vi "Copy Raw Data.vi"(8 "error in (no error)":errorcluster, 10 "new tdms file":refnum<k34>, 11 "original tdms file":refnum<k34>) -> (0 "error out":errorcluster, 3 "dup original tdms file":refnum<k34>)   [LabVIEW 2023]
doc: "Read raw data out from original file using standard read and write it to the new file with advanced synchronous write"
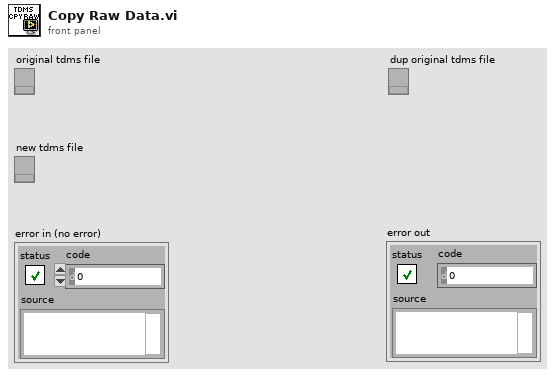
[diagram p1: front panel]
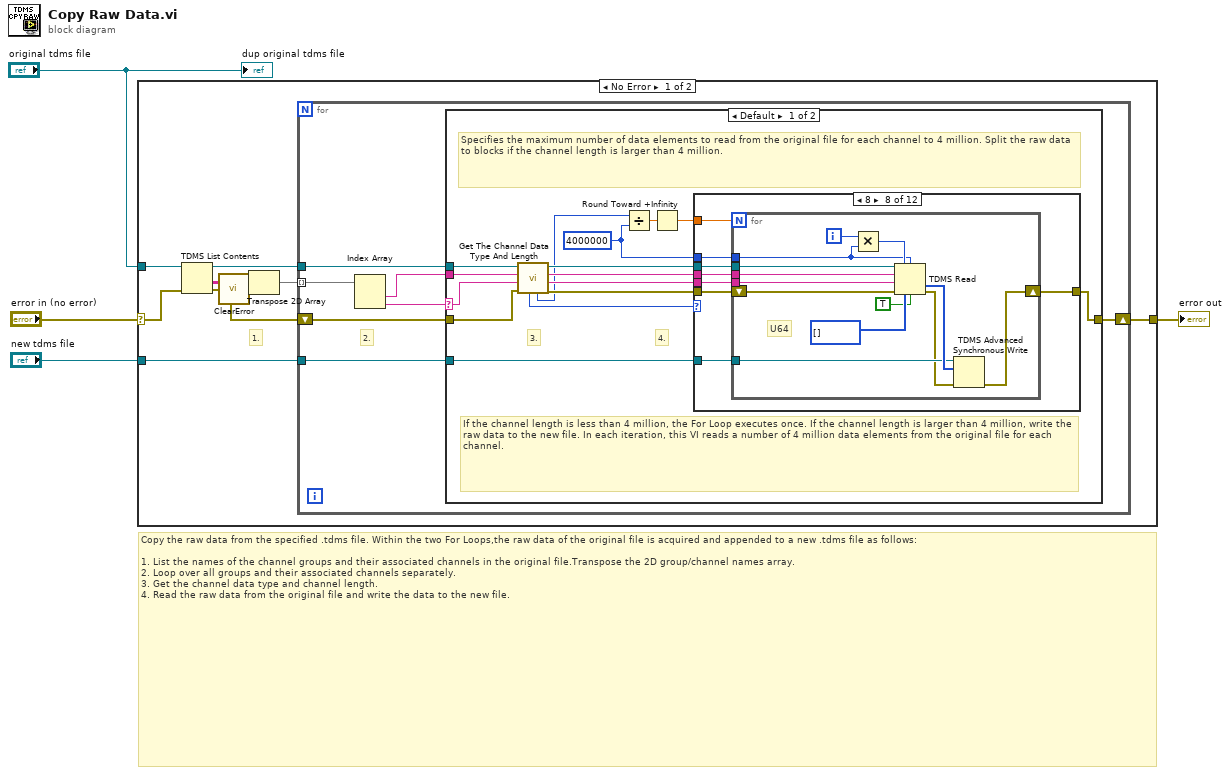
[diagram p0: block diagram]
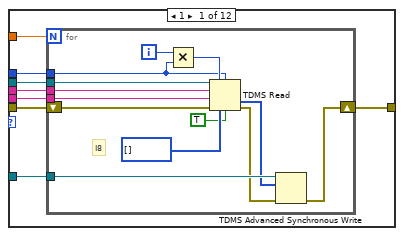
[diagram p2: hidden frame]
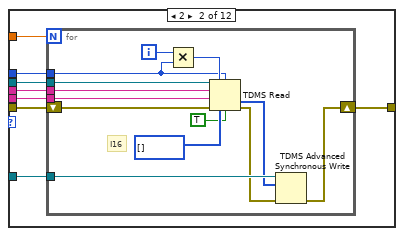
[diagram p3: hidden frame]
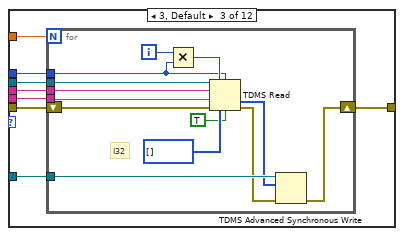
[diagram p4: hidden frame]
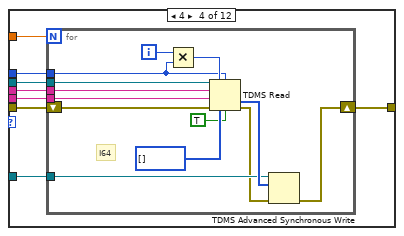
[diagram p5: hidden frame]
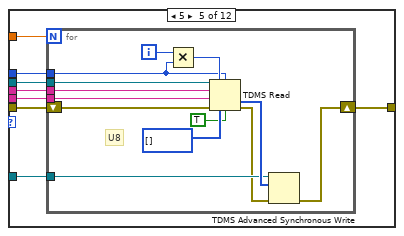
[diagram p6: hidden frame]
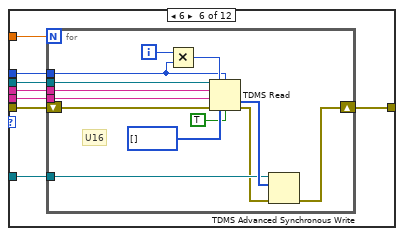
[diagram p7: hidden frame]
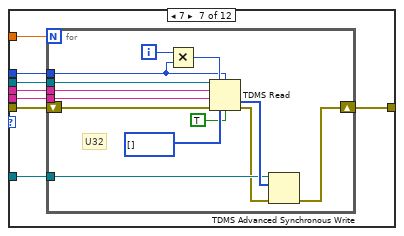
[diagram p8: hidden frame]
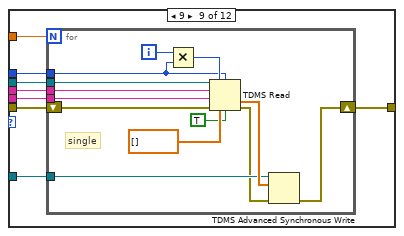
[diagram p9: hidden frame]
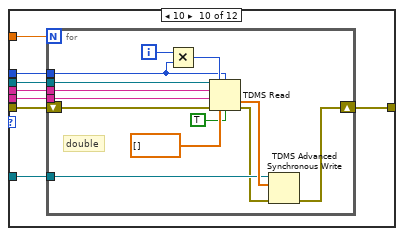
[diagram p10: hidden frame]
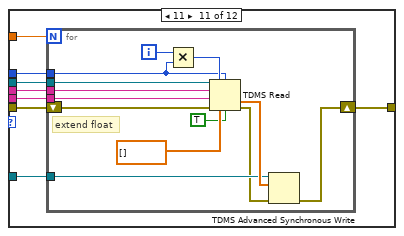
[diagram p11: hidden frame]
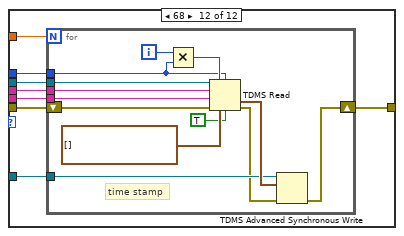
[diagram p12: hidden frame]
diagram:
  # "Copy the raw data from the specified .tdms file. Within the two For Loops,the raw data of the original file is acquired and appended to a new .tdms file as follows:\n\n1. List the names of the channel groups and their associated channels in the original file.Transpose the 2D group/channel names array.\n2. Loop over all groups and their associated channels separately.\n3. Get the channel data type and channel length.\n4. Read the raw data from the original file and write the data to the new file."
  n1 = case shown="No Error" "error in (no error)" {
    selector: "error in (no error)" -> [w7 w289]
    tunnel: "new tdms file" -> [w13 _]
    tunnel: [w12 w289] -> w2
    tunnel: "original tdms file" -> [w9 _]
    frame No Error {
      # "1."
      n2 = TDMS List Contents(4:w7, 7:w9) -> (0:w5:errorcluster, 1:w10:string[][], 3:w8:refnum<k34>)  [unwired: 1 in, 1 out]
      n3 = call <vilib>:"ClearError.vi"("error in (no error)"=w5) -> ("error out"=w6:errorcluster)
      n4 = Transpose 2D Array(2D array=w10) -> (transposed array=w11:string[][])
      n5 = for {
        shift-right: [w17] -> w12
        shift-left: w6 -> [w18]
        tunnel: w11 -> [w15] mode=indexing
        tunnel: w8 -> [w20]
        tunnel: w13 -> [w19]
        # "2."
        n6 = Index Array(array=w15) -> (element #1=w16:string, element #2=w14:string)  [unwired: 2 in]
        n7 = case shown="Default" w14 {
          selector: w14 -> [w21 _]
          tunnel: w20 -> [w35 _]
          tunnel: w19 -> [w34 _]
          tunnel: w18 -> [w33 w288]
          tunnel: [w31 w288] -> w17
          tunnel: w16 -> [w26 _]
          frame Default {
            w24 = 4000000 ("y")
            # "If the channel length is less than 4 million, the For Loop executes once. If the channel length is larger than 4 million, write the raw data to the new file. In each iteration, this VI reads a number of 4 million data elements from the original file for each channel."
            # "Specifies the maximum number of data elements to read from the original file for each channel to 4 million. Split the raw data to blocks if the channel length is larger than 4 million."
            # "4."
            # "3."
            n8 = call "Get The Channel Data Type And Length.vi"("error in (no error)"=w33, "channel name"=w21, "group name"=w26, "tdms file"=w35) -> ("error out"=w32:errorcluster, "dup channel name"=w27:string, "dup group name"=w28:string, "dup tdms file"=w30:refnum<k34>, "channel length"=w25:i32, "data type"=w29:i32)  [unwired: 2 in]
            n9 = Divide(x=w25, y=w24) -> (x/y=w23:dbl)
            n10 = Round Toward +Infinity(x=w23) -> (ceil(x): smallest int >= x=w22:dbl)
            n11 = case shown="8" w29 {
              tunnel: w30 -> [w41 w62 w83 w104 w125 w146 w167 w188 w209 w230 w251 w272]
              tunnel: w34 -> [w40 w61 w82 w103 w124 w145 w166 w187 w208 w229 w250 w271]
              tunnel: w28 -> [w39 w60 w81 w102 w123 w144 w165 w186 w207 w228 w249 w270]
              tunnel: w27 -> [w38 w59 w80 w101 w122 w143 w164 w185 w206 w227 w248 w269]
              tunnel: w22 -> [w43 w64 w85 w106 w127 w148 w169 w190 w211 w232 w253 w274]
              tunnel: w24 -> [w42 w63 w84 w105 w126 w147 w168 w189 w210 w231 w252 w273]
              tunnel: w32 -> [w37 w58 w79 w100 w121 w142 w163 w184 w205 w226 w247 w268]
              tunnel: [w36 w57 w78 w99 w120 w141 w162 w183 w204 w225 w246 w267] -> w31
              frame 1 {
                n12 = for {
                  N: w43 -> [_]
                  tunnel: w42 -> [w47]
                  tunnel: w39 -> [w53]
                  tunnel: w38 -> [w52]
                  shift-right: [w48] -> w36
                  shift-left: w37 -> [w50]
                  tunnel: w41 -> [w55]
                  tunnel: w40 -> [w54]
                  i -> [w51]
                  # "I8"
                  n13 = Multiply(x=w51, y=w47) -> (x*y=w56:i32)
                  n14 = TDMS Read(0:w55, 1:w56, 2:w47, 5:w53, 7:w52, 11:w50, 12:i8[] [], 13:TRUE ("return channels in file order? (F)")) -> (10:w46:i8[], 15:w49:errorcluster)  [unwired: 4 out]
                  n15 = TDMS Advanced Synchronous Write(8:w49, 10:w46, 11:w54) -> (0:w48:errorcluster)  [unwired: 1 out]
                }
              }
              frame 2 {
                n16 = for {
                  N: w64 -> [_]
                  tunnel: w63 -> [w68]
                  tunnel: w60 -> [w74]
                  tunnel: w59 -> [w73]
                  shift-right: [w69] -> w57
                  shift-left: w58 -> [w71]
                  tunnel: w62 -> [w76]
                  tunnel: w61 -> [w75]
                  i -> [w72]
                  # "I16"
                  n17 = Multiply(x=w72, y=w68) -> (x*y=w77:i32)
                  n18 = TDMS Read(0:w76, 1:w77, 2:w68, 5:w74, 7:w73, 11:w71, 12:i16[] [], 13:TRUE ("return channels in file order? (F)")) -> (10:w67:i16[], 15:w70:errorcluster)  [unwired: 4 out]
                  n19 = TDMS Advanced Synchronous Write(8:w70, 10:w67, 11:w75) -> (0:w69:errorcluster)  [unwired: 1 out]
                }
              }
              frame 3, Default {
                n20 = for {
                  N: w85 -> [_]
                  tunnel: w84 -> [w89]
                  tunnel: w81 -> [w95]
                  tunnel: w80 -> [w94]
                  shift-right: [w90] -> w78
                  shift-left: w79 -> [w92]
                  tunnel: w83 -> [w97]
                  tunnel: w82 -> [w96]
                  i -> [w93]
                  # "I32"
                  n21 = Multiply(x=w93, y=w89) -> (x*y=w98:i32)
                  n22 = TDMS Read(0:w97, 1:w98, 2:w89, 5:w95, 7:w94, 11:w92, 12:i32[] [], 13:TRUE ("return channels in file order? (F)")) -> (10:w88:i32[], 15:w91:errorcluster)  [unwired: 4 out]
                  n23 = TDMS Advanced Synchronous Write(8:w91, 10:w88, 11:w96) -> (0:w90:errorcluster)  [unwired: 1 out]
                }
              }
              frame 4 {
                n24 = for {
                  N: w106 -> [_]
                  tunnel: w105 -> [w109]
                  tunnel: w102 -> [w115]
                  tunnel: w101 -> [w114]
                  shift-right: [w110] -> w99
                  shift-left: w100 -> [w112]
                  tunnel: w104 -> [w117]
                  tunnel: w103 -> [w116]
                  i -> [w113]
                  # "I64"
                  n25 = Multiply(x=w113, y=w109) -> (x*y=w118:i32)
                  n26 = TDMS Read(0:w117, 1:w118, 2:w109, 5:w115, 7:w114, 11:w112, 12:i64[] [], 13:TRUE ("return channels in file order? (F)")) -> (10:w119:i64[], 15:w111:errorcluster)  [unwired: 4 out]
                  n27 = TDMS Advanced Synchronous Write(8:w111, 10:w119, 11:w116) -> (0:w110:errorcluster)  [unwired: 1 out]
                }
              }
              frame 5 {
                n28 = for {
                  N: w127 -> [_]
                  tunnel: w126 -> [w130]
                  tunnel: w123 -> [w136]
                  tunnel: w122 -> [w135]
                  shift-right: [w131] -> w120
                  shift-left: w121 -> [w133]
                  tunnel: w125 -> [w138]
                  tunnel: w124 -> [w137]
                  i -> [w134]
                  # "U8"
                  n29 = Multiply(x=w134, y=w130) -> (x*y=w139:i32)
                  n30 = TDMS Read(0:w138, 1:w139, 2:w130, 5:w136, 7:w135, 11:w133, 12:u8[] [], 13:TRUE ("return channels in file order? (F)")) -> (10:w140:u8[], 15:w132:errorcluster)  [unwired: 4 out]
                  n31 = TDMS Advanced Synchronous Write(8:w132, 10:w140, 11:w137) -> (0:w131:errorcluster)  [unwired: 1 out]
                }
              }
              frame 6 {
                n32 = for {
                  N: w148 -> [_]
                  tunnel: w147 -> [w151]
                  tunnel: w144 -> [w157]
                  tunnel: w143 -> [w156]
                  shift-right: [w152] -> w141
                  shift-left: w142 -> [w154]
                  tunnel: w146 -> [w159]
                  tunnel: w145 -> [w158]
                  i -> [w155]
                  # "U16"
                  n33 = Multiply(x=w155, y=w151) -> (x*y=w160:i32)
                  n34 = TDMS Read(0:w159, 1:w160, 2:w151, 5:w157, 7:w156, 11:w154, 12:u16[] [], 13:TRUE ("return channels in file order? (F)")) -> (10:w161:u16[], 15:w153:errorcluster)  [unwired: 4 out]
                  n35 = TDMS Advanced Synchronous Write(8:w153, 10:w161, 11:w158) -> (0:w152:errorcluster)  [unwired: 1 out]
                }
              }
              frame 7 {
                n36 = for {
                  N: w169 -> [_]
                  tunnel: w168 -> [w172]
                  tunnel: w165 -> [w178]
                  tunnel: w164 -> [w177]
                  shift-right: [w173] -> w162
                  shift-left: w163 -> [w175]
                  tunnel: w167 -> [w180]
                  tunnel: w166 -> [w179]
                  i -> [w176]
                  # "U32"
                  n37 = Multiply(x=w176, y=w172) -> (x*y=w181:i32)
                  n38 = TDMS Read(0:w180, 1:w181, 2:w172, 5:w178, 7:w177, 11:w175, 12:u32[] [], 13:TRUE ("return channels in file order? (F)")) -> (10:w182:u32[], 15:w174:errorcluster)  [unwired: 4 out]
                  n39 = TDMS Advanced Synchronous Write(8:w174, 10:w182, 11:w179) -> (0:w173:errorcluster)  [unwired: 1 out]
                }
              }
              frame 8 {
                n40 = for {
                  N: w190 -> [_]
                  tunnel: w189 -> [w193]
                  tunnel: w186 -> [w199]
                  tunnel: w185 -> [w198]
                  shift-right: [w194] -> w183
                  shift-left: w184 -> [w196]
                  tunnel: w188 -> [w201]
                  tunnel: w187 -> [w200]
                  i -> [w197]
                  # "U64"
                  n41 = Multiply(x=w197, y=w193) -> (x*y=w202:i32)
                  n42 = TDMS Read(0:w201, 1:w202, 2:w193, 5:w199, 7:w198, 11:w196, 12:u64[] [], 13:TRUE ("return channels in file order? (F)")) -> (10:w203:u64[], 15:w195:errorcluster)  [unwired: 4 out]
                  n43 = TDMS Advanced Synchronous Write(8:w195, 10:w203, 11:w200) -> (0:w194:errorcluster)  [unwired: 1 out]
                }
              }
              frame 9 {
                n44 = for {
                  N: w211 -> [_]
                  tunnel: w210 -> [w214]
                  tunnel: w207 -> [w220]
                  tunnel: w206 -> [w219]
                  shift-right: [w215] -> w204
                  shift-left: w205 -> [w217]
                  tunnel: w209 -> [w222]
                  tunnel: w208 -> [w221]
                  i -> [w218]
                  # "single"
                  n45 = Multiply(x=w218, y=w214) -> (x*y=w223:i32)
                  n46 = TDMS Read(0:w222, 1:w223, 2:w214, 5:w220, 7:w219, 11:w217, 12:sgl[] [], 13:TRUE ("return channels in file order? (F)")) -> (10:w224:sgl[], 15:w216:errorcluster)  [unwired: 4 out]
                  n47 = TDMS Advanced Synchronous Write(8:w216, 10:w224, 11:w221) -> (0:w215:errorcluster)  [unwired: 1 out]
                }
              }
              frame 10 {
                n48 = for {
                  N: w232 -> [_]
                  tunnel: w231 -> [w235]
                  tunnel: w228 -> [w241]
                  tunnel: w227 -> [w240]
                  shift-right: [w236] -> w225
                  shift-left: w226 -> [w238]
                  tunnel: w230 -> [w243]
                  tunnel: w229 -> [w242]
                  i -> [w239]
                  # "double"
                  n49 = Multiply(x=w239, y=w235) -> (x*y=w244:i32)
                  n50 = TDMS Read(0:w243, 1:w244, 2:w235, 5:w241, 7:w240, 11:w238, 12:dbl[] [], 13:TRUE ("return channels in file order? (F)")) -> (10:w245:dbl[], 15:w237:errorcluster)  [unwired: 4 out]
                  n51 = TDMS Advanced Synchronous Write(8:w237, 10:w245, 11:w242) -> (0:w236:errorcluster)  [unwired: 1 out]
                }
              }
              frame 11 {
                n52 = for {
                  N: w253 -> [_]
                  tunnel: w252 -> [w256]
                  tunnel: w249 -> [w262]
                  tunnel: w248 -> [w261]
                  shift-right: [w257] -> w246
                  shift-left: w247 -> [w259]
                  tunnel: w251 -> [w264]
                  tunnel: w250 -> [w263]
                  i -> [w260]
                  # "extend float"
                  n53 = Multiply(x=w260, y=w256) -> (x*y=w265:i32)
                  n54 = TDMS Read(0:w264, 1:w265, 2:w256, 5:w262, 7:w261, 11:w259, 12:ext[] [], 13:TRUE ("return channels in file order? (F)")) -> (10:w266:ext[], 15:w258:errorcluster)  [unwired: 4 out]
                  n55 = TDMS Advanced Synchronous Write(8:w258, 10:w266, 11:w263) -> (0:w257:errorcluster)  [unwired: 1 out]
                }
              }
              frame 68 {
                n56 = for {
                  N: w274 -> [_]
                  tunnel: w273 -> [w277]
                  tunnel: w270 -> [w283]
                  tunnel: w269 -> [w282]
                  shift-right: [w278] -> w267
                  shift-left: w268 -> [w280]
                  tunnel: w272 -> [w285]
                  tunnel: w271 -> [w284]
                  i -> [w281]
                  # "time stamp"
                  n57 = Multiply(x=w281, y=w277) -> (x*y=w286:i32)
                  n58 = TDMS Read(0:w285, 1:w286, 2:w277, 5:w283, 7:w282, 11:w280, 12:timestamp[] [], 13:TRUE ("return channels in file order? (F)")) -> (10:w287:timestamp[], 15:w279:errorcluster)  [unwired: 4 out]
                  n59 = TDMS Advanced Synchronous Write(8:w279, 10:w287, 11:w284) -> (0:w278:errorcluster)  [unwired: 1 out]
                }
              }
            }
          }
          frame "" {
            # "If the group has no channels, do nothing."
          }
        }
      }
    }
    frame Error {
    }
  }
  "error out" <- w2
  "dup original tdms file" <- "original tdms file"
